vi "GP22_TDC_Arduinoed Single Measurement.vi"() -> ()   [LabVIEW 2014, in "GP22_TDC_Arduinoed.lvlib"]
uses:
  GP22_TDC_Arduinoed.lvlib
panel:
  out "output":dbl format="%^#_6g"
  out "Freq / Hz":dbl
  out "error out":errorcluster
  out "Self-Test Result Message":string
  in  "VISA resource name":refnum<visa-resource-name>
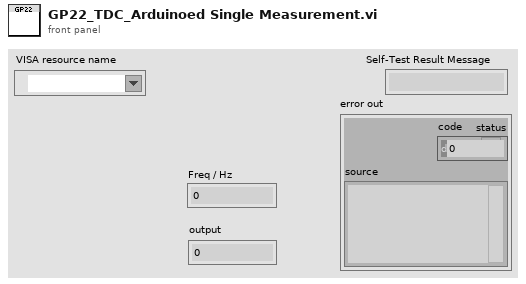
[diagram p1: front panel]
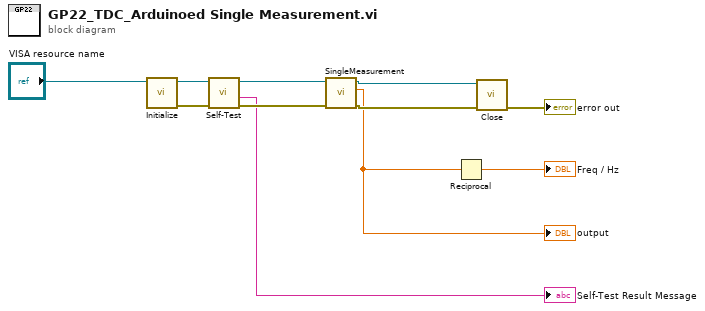
[diagram p0: block diagram]
diagram:
  n1 = call "Initialize.vi"("VISA resource name"="VISA resource name") -> ("error out"=w6:errorcluster, "VISA resource name out"=w9:refnum<visa-resource-name>)  [unwired: 9 in]
  n2 = call "Self-Test.vi"("error in (no error)"=w6, "VISA resource name"=w9) -> ("error out"=w7:errorcluster, "Self-Test Result Message"=→"Self-Test Result Message":string, "VISA resource name out"=w8:refnum<visa-resource-name>)  [unwired: 6 in, 1 out]
  n3 = call "SingleMeasurement.vi"("VISA resource name"=w8) -> ("output"=w1:dbl, "VISA resource name out"=w3:refnum<visa-resource-name>)  [unwired: 8 in, 1 out]
  "output" <- w1
  n4 = Reciprocal(x=w1) -> (1/x=→"Freq / Hz":dbl)
  n5 = call "Close.vi"("error in (no error)"=w7, "VISA resource name"=w3) -> ("error out"=→"error out":errorcluster)  [unwired: 9 in]
